vi "FPGA Main.vi"() -> ()   [LabVIEW 2021]
uses:
  <vilib>/rvi/Emulation/niFpgaGetClockAttributes.vi
  <vilib>/rvi/Emulation/niFpgaSctlEmulationGetInTimedLoop.vi
  <vilib>/rvi/Emulation/niFpgaEmulationReportErrorSimple.vi
  <vilib>/rvi/eio/common/nirviEmuTemplateMethod_errors.vi
  <vilib>/rvi/Emulation/niFpgaCriticalErrorInLSC.vi
  <vilib>/eio/EIONode/EIONode.xnode
panel:
  out "Chassis Temperature":i16
  in  "Boolean":bool
  in  "U64 Value":u64
  out "U64 Out":u64
  out "U32 Out":u32
  in  "U32 Value":u32
  out "U16 Out":u16
  in  "U16 Value":u16
  out "U8 Out":u8
  in  "U8 Value":u8
  in  "I8 Value":i8
  out "I8 Out":i8
  in  "I16 Value":i16
  out "I16 Out":i16
  in  "I32 Value":i32
  out "I32 Out":i32
  in  "I64 Value":i64
  out "I64 Out":i64
  out "Single Out":sgl
  in  "Single Value":sgl
  in  "Mod2/DIO3":bool
  in  "Mod2/DIO2":bool
  out "Mod2/DIO1":bool
  out "Mod2/DIO0":bool
  in  "Mod2/AO7":fxp<+,16,3>
  in  "Mod2/AO6":fxp<+,16,3>
  in  "Mod2/AO5":fxp<+,16,3>
  in  "Mod2/AO4":fxp<+,16,3>
  in  "Mod2/AO3":fxp<+,16,3>
  in  "Mod2/AO2":fxp<+,16,3>
  in  "Mod2/AO1":fxp<+,16,3>
  in  "Mod2/AO0":fxp<+,16,3>
  out "Mod2/AI7":fxp<+,18,3>
  out "Mod2/AI6":fxp<+,18,3>
  out "Mod2/AI5":fxp<+,18,3>
  out "Mod2/AI4":fxp<+,18,3>
  out "Mod2/AI3":fxp<+,18,3>
  out "Mod2/AI2":fxp<+,18,3>
  out "Mod2/AI1":fxp<+,18,3>
  out "Mod2/AI0":fxp<+,18,3>
  out "Mod1/Autozero":fxp<+/-,24,-2>
  out "Mod1/CJC":fxp<+/-,24,-2>
  out "Mod1/TC3":fxp<+/-,24,-2>
  out "Mod1/TC2":fxp<+/-,24,-2>
  out "Mod1/TC1":fxp<+/-,24,-2>
  out "Mod1/TC0":fxp<+/-,24,-2>
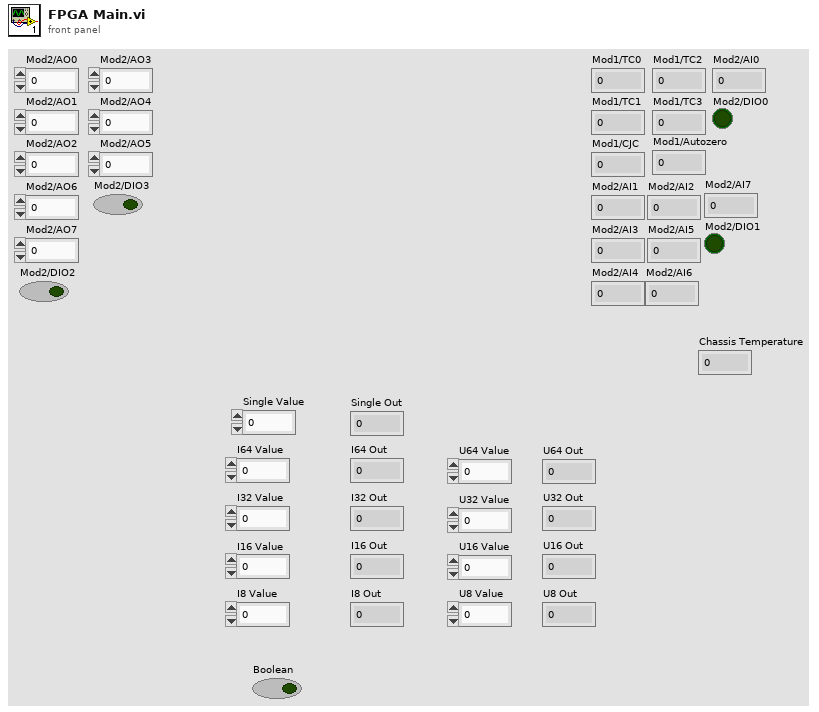
[diagram p1: front panel]
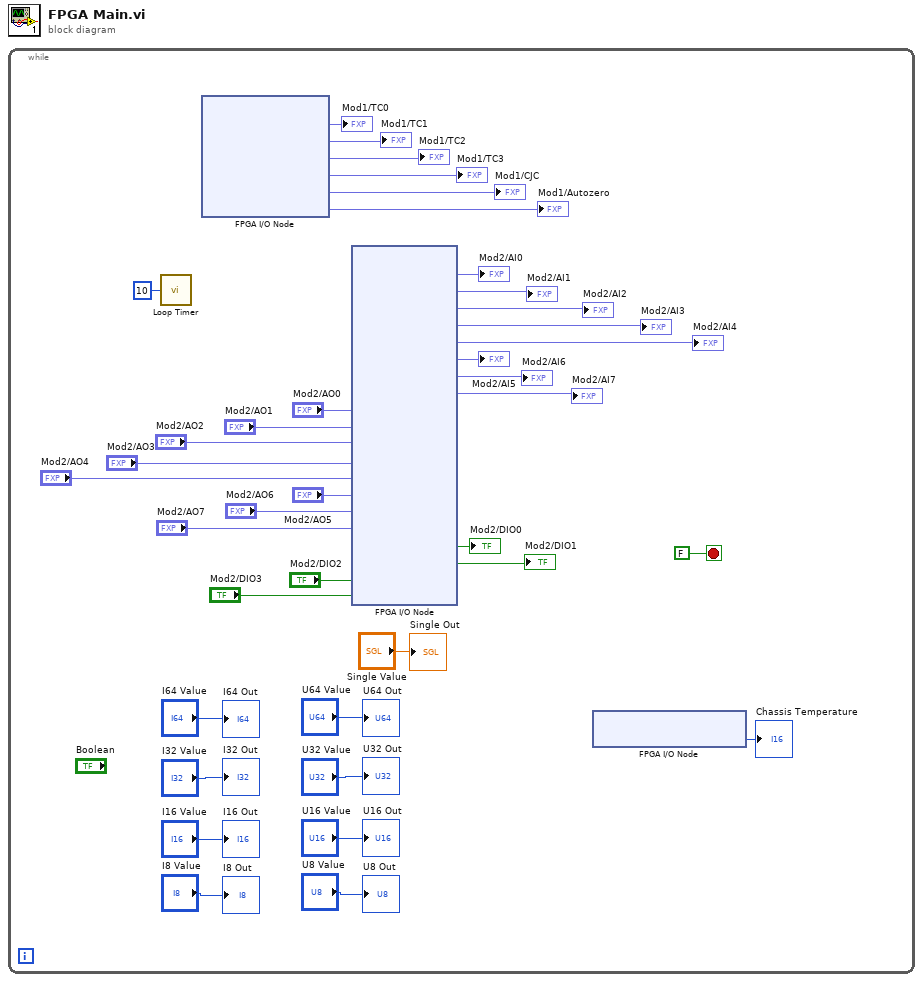
[diagram p0: block diagram]
diagram:
  n1 = while {
    stop <- FALSE stop-if-true
    n2 = call "Loop Timer"("Count(mSec)"=u32 10) -> ()  [unwired: 1 out]
    n3 = xnode "FPGA I/O Node"() -> ("Mod1/TC0"=→"Mod1/TC0":fxp<+/-,24,-2>, "Mod1/TC1"=→"Mod1/TC1":fxp<+/-,24,-2>, "Mod1/TC2"=→"Mod1/TC2":fxp<+/-,24,-2>, "Mod1/TC3"=→"Mod1/TC3":fxp<+/-,24,-2>, "Mod1/CJC"=→"Mod1/CJC":fxp<+/-,24,-2>, "Mod1/Autozero"=→"Mod1/Autozero":fxp<+/-,24,-2>)  [unwired: 6 in, 6 out]
    n4 = xnode "FPGA I/O Node"("Mod2/AO0"="Mod2/AO0", "Mod2/AO1"="Mod2/AO1", "Mod2/AO2"="Mod2/AO2", "Mod2/AO3"="Mod2/AO3", "Mod2/AO4"="Mod2/AO4", "Mod2/AO5"="Mod2/AO5", "Mod2/AO6"="Mod2/AO6", "Mod2/AO7"="Mod2/AO7", "Mod2/DIO2"="Mod2/DIO2", "Mod2/DIO3"="Mod2/DIO3") -> ("Mod2/AI0"=→"Mod2/AI0":fxp<+,18,3>, "Mod2/AI1"=→"Mod2/AI1":fxp<+,18,3>, "Mod2/AI2"=→"Mod2/AI2":fxp<+,18,3>, "Mod2/AI3"=→"Mod2/AI3":fxp<+,18,3>, "Mod2/AI4"=→"Mod2/AI4":fxp<+,18,3>, "Mod2/AI5"=→"Mod2/AI5":fxp<+,18,3>, "Mod2/AI6"=→"Mod2/AI6":fxp<+,18,3>, "Mod2/AI7"=→"Mod2/AI7":fxp<+,18,3>, "Mod2/DIO0"=→"Mod2/DIO0":bool, "Mod2/DIO1"=→"Mod2/DIO1":bool)  [unwired: 20 in, 20 out]
    n5 = xnode "FPGA I/O Node"() -> ("Chassis Temperature"=→"Chassis Temperature":i16)  [unwired: 1 in, 1 out]
    "Single Out" <- "Single Value"
    "I64 Out" <- "I64 Value"
    "I32 Out" <- "I32 Value"
    "I16 Out" <- "I16 Value"
    "I8 Out" <- "I8 Value"
    "U64 Out" <- "U64 Value"
    "U32 Out" <- "U32 Value"
    "U16 Out" <- "U16 Value"
    "U8 Out" <- "U8 Value"
  }
